vi "Calculate Angle.vi"(9 "Normalized.Rectangle":T1, 10 "Goal Display":T2(plugin-control)) -> (2 "Angle Difference":dbl)   [LabVIEW 2016]
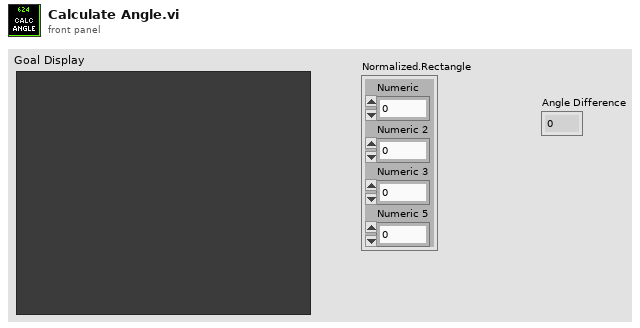
[diagram p1: front panel]
types:
  T1 = cluster{"Numeric":dbl, "Numeric 2":dbl, "Numeric 3":dbl, "Numeric 5":dbl}
  T2 = typedef "IMAQ Image.ctl" = refnum<image>
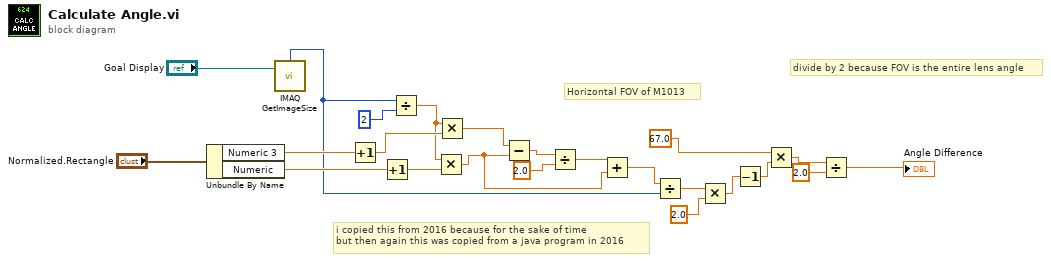
[diagram p0: block diagram]
diagram:
  # "i copied this from 2016 because for the sake of time\nbut then again this was copied from a java program in 2016"
  # "divide by 2 because FOV is the entire lens angle"
  # "Horizontal FOV of M1013"
  n1 = Unbundle By Name("Normalized.Rectangle") -> ("Numeric 3"=w20:dbl, "Numeric"=w17:dbl)
  n2 = call "IMAQ GetImageSize"("Image"="Goal Display") -> ("X Resolution"=w10:i32)  [unwired: 3 in, 2 out]
  n3 = Increment(x=w20) -> (x+1=w19:dbl)
  n4 = Increment(x=w17) -> (x+1=w16:dbl)
  n5 = Divide(x=w10, y=2) -> (x/y=w18:dbl)
  n6 = Multiply(x=w18, y=w16) -> (x*y=w11:dbl)
  n7 = Multiply(x=w18, y=w19) -> (x*y=w15:dbl)
  n8 = Subtract(x=w15, y=w11) -> (x-y=w14:dbl)
  n9 = Divide(x=w14, y=2.0) -> (x/y=w12:dbl)
  n10 = Add(x=w12, y=w11) -> (x+y=w9:dbl)
  n11 = Divide(x=w9, y=w10) -> (x/y=w8:dbl)
  n12 = Multiply(x=w8, y=2.0) -> (x*y=w6:dbl)
  n13 = Decrement(x=w6) -> (x-1=w5:dbl)
  n14 = Multiply(x=67.0, y=w5) -> (x*y=w3:dbl)
  n15 = Divide(x=w3, y=2.0) -> (x/y=→"Angle Difference":dbl)
